vi "Autonomous Independent.vi"   [LabVIEW 2018]
doc: "This VI is called when autonomous begins, and will automatically be terminated when autonomous ends. You can carry out timed or sensor driven robot movement independently without needing to return to the caller."
uses:
  <vilib>/Rock Robotics/WPI/Utilities/WPI_GetSetVariantRefNum.vi
  <vilib>/Rock Robotics/Network Tables/NT Read String.vi
  Robot Global Data.vi
  <vilib>/Rock Robotics/WPI/RobotDrive/WPI_RobotDriveMecanumDrive_Cartesian.vi
panel:
  # "Be sure to right-click and choose Data Operations>>Make Current Value default if you want to save the array values with the VI"
types:
  T1 = typedef "WPI_RobotDriveDevRef.ctl" = cluster{"DevStatus":errorcluster, "Motors[]":T2[], "Square Inputs":bool, "Max Output":dbl}
  T2 = typedef "WPI_MotorControlDeviceRef.ctl" = cluster{"DeviceStatus":errorcluster, "Type":T3, "PWM":cluster{"PWM Channel":T4, "DeadBand":T5}, "CAN":cluster{"Device Number":u8, "SetOutput VI Ref":variant, "GetOutput VI Ref":variant, "Enable VI Ref":variant, "Disable VI Ref":variant, "Data":variant}, "Invert":bool, "DIO PWM":cluster{"PWM \"Enable\" Channel":T4, "DIOChannel":T6, "PWM Rate":dbl}}
  T3 = typedef "WPI_MotorControlType.ctl" = enum16{"PWM", "CAN", "DIO PWM"}
  T4 = typedef "FPGA_DIOPWMChannel.ctl" = enum8{"PWM 0", "PWM 1", "PWM 2", "PWM 3", "PWM 4", "PWM 5", "PWM 6", "PWM 7", "PWM 8", "PWM 9", "PWM MXP 0", "PWM MXP 1", "PWM MXP 2", "PWM MXP 3", "PWM MXP 4", "PWM MXP 5", "PWM MXP 6", "PWM MXP 7", "PWM MXP 8", "PWM MXP 9", "Invalid"}
  T5 = typedef "WPI_PWMDeadband.ctl" = cluster{"Name":string, "maxPositivePwm":i32, "minPositivePwm":i32, "centerPwm":i32, "maxNegativePwm":i32, "minNegativePwm":i32, "angularRange":u16}
  T6 = typedef "FPGA_DIOChannel.ctl" = enum8{"DIO 0", "DIO 1", "DIO 2", "DIO 3", "DIO 4", "DIO 5", "DIO 6", "DIO 7", "DIO 8", "DIO 9", "DIO MXP 0", "DIO MXP 1", "DIO MXP 2", "DIO MXP 3", "DIO MXP 4", "DIO MXP 5", "DIO MXP 6", "DIO MXP 7", "DIO MXP 8", "DIO MXP 9", "DIO MXP 10", "DIO MXP 11", "DIO MXP 12", "DIO MXP 13", "DIO MXP 14", "DIO MXP 15", "SPI Port CS1", "SPI Port CS2", "SPI Port CS3", "SPI Port MISO", "SPI Port MOSI", "Invalid"}
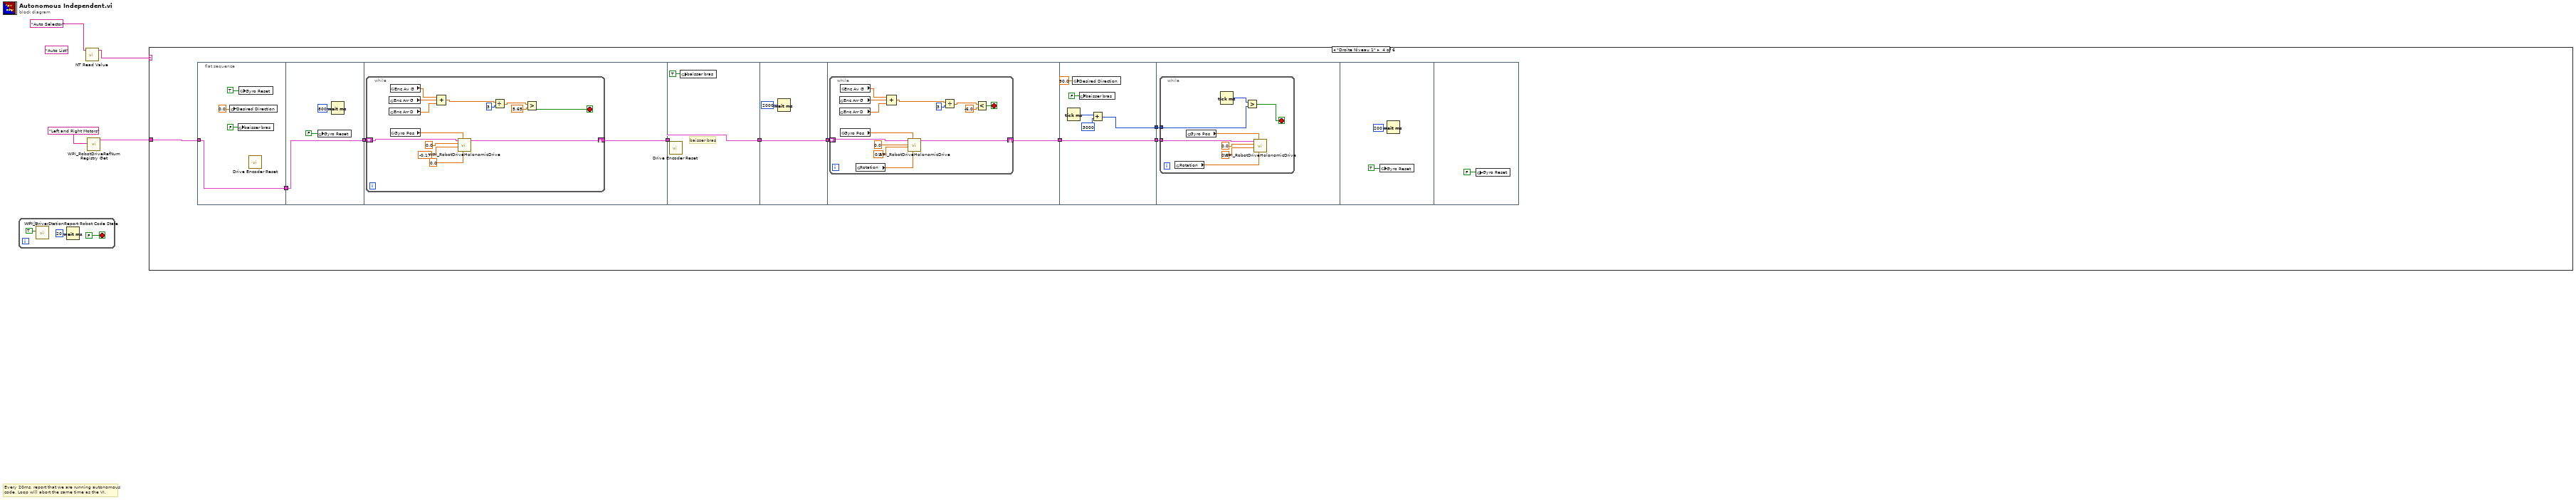
[diagram p0: block diagram]
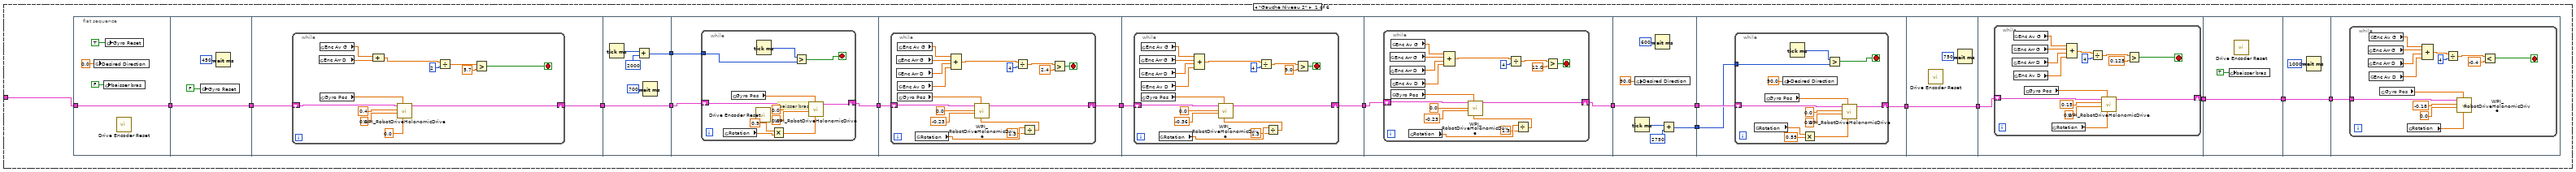
[diagram p2: hidden frame]
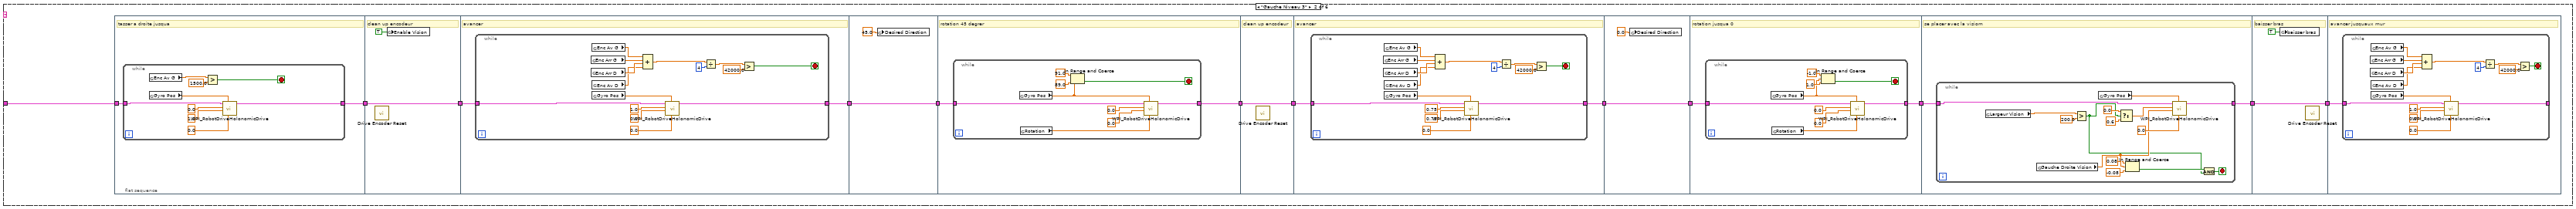
[diagram p3: hidden frame]
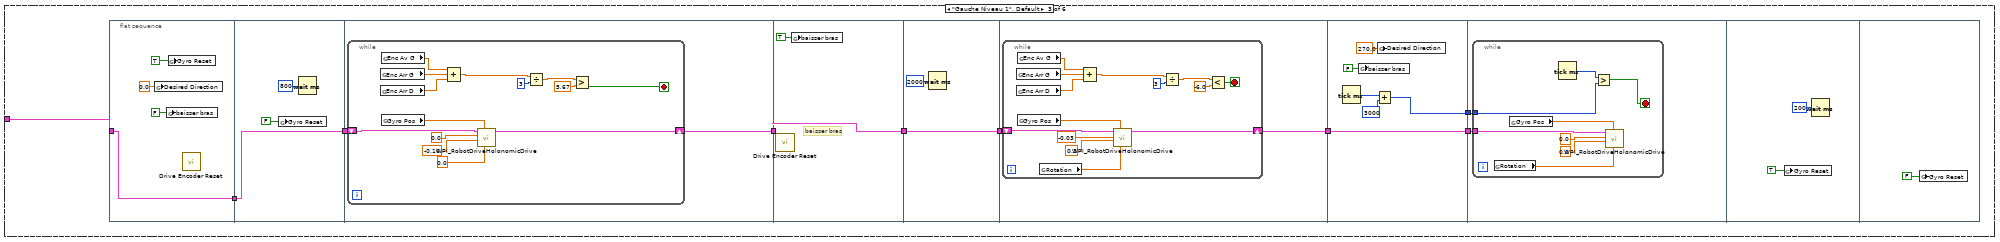
[diagram p4: hidden frame]
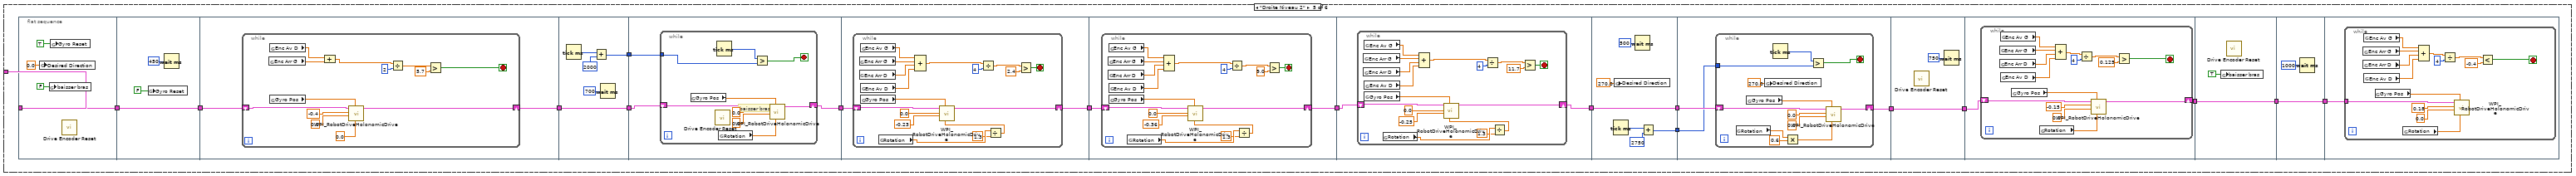
[diagram p5: hidden frame]
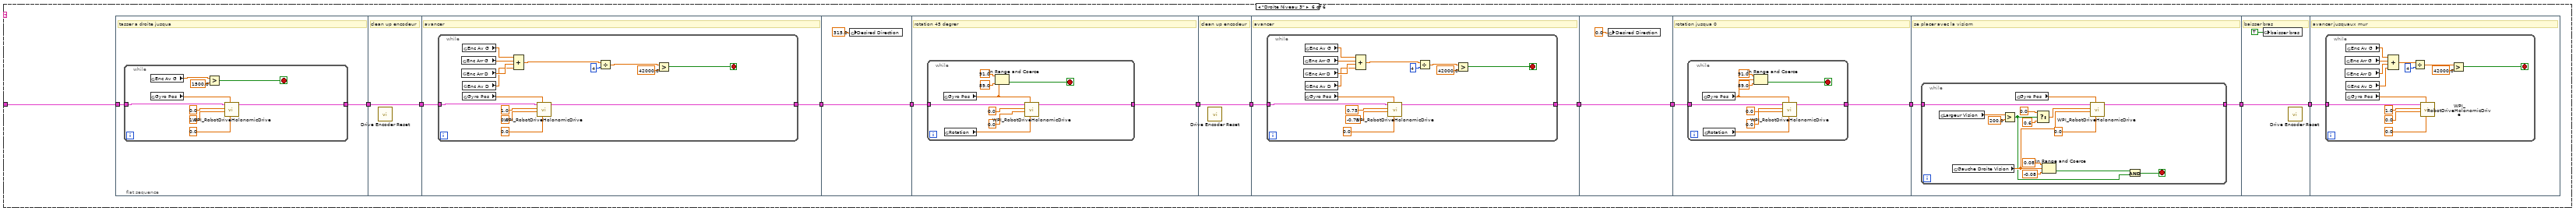
[diagram p6: hidden frame]
diagram:
  (unwired) "Auto List" ("Name")
  # "Every 20ms, report that we are running autonomous\ncode. Loop will abort the same time as the VI."
  n1 = while {
    stop <- FALSE stop-if-true
    n2 = call <vilib>:"WPI_DriverStationReport Robot Code State.vi"("Autonomous"=TRUE) -> ()  [unwired: 10 in, 1 out]
    n3 = Wait (ms)(milliseconds to wait=u32 20) -> ()  [unwired: 1 out]
  }
  n4 = call-poly <vilib>:"NT Read Value.vi"("Name"="Auto Selector") -> ("String"=w4:string)  [unwired: 9 in, 1 out]
  n5 = call <vilib>:"WPI_RobotDriveRefNum Registry Get.vi"("refnum name"="Left and Right Motors") -> ("RobotDriveDevRef"=w2:T1)  [unwired: 1 in, 9 out]
  n6 = case shown="\"Droite Niveau 1\"" w4 {
    tunnel: w2 -> [w8 w189 w303 w381 w459 w617]
    frame "Gauche Niveau 2" {
      n7 = flat-sequence {
        tunnel: w8 -> [w28]
        tunnel: [w28] -> w24
        tunnel: w24 -> [w29]
        tunnel: [w29] -> w23
        tunnel: [w33] -> w22
        tunnel: w23 -> [w32]
        tunnel: w22 -> [w51]
        tunnel: [w51] -> w21
        tunnel: [w48] -> w20
        tunnel: [w53] -> w19
        tunnel: w21 -> [w54]
        tunnel: w20 -> [w52]
        tunnel: w19 -> [w67]
        tunnel: [w66] -> w18
        tunnel: w18 -> [w86]
        tunnel: [w85] -> w17
        tunnel: w17 -> [w105]
        tunnel: [w104] -> w16
        tunnel: [w127] -> w15
        tunnel: w16 -> [w127]
        tunnel: [w123] -> w14
        tunnel: w15 -> [w131]
        tunnel: [w130] -> w13
        tunnel: w14 -> [w129]
        tunnel: w13 -> [w145]
        tunnel: [w145] -> w12
        tunnel: w12 -> [w147]
        tunnel: [w146] -> w11
        tunnel: w11 -> [w163]
        tunnel: [w163] -> w10
        tunnel: w10 -> [w166]
        tunnel: [w166] -> w9
        tunnel: w9 -> [w167]
        frame #0 {
          n8 = global write "Robot Global Data.vi" "Desired Direction"(0.0 ("Desired Direction")) -> ()
          n9 = global write "Robot Global Data.vi" "baisser bras"(FALSE) -> ()
          n10 = global write "Robot Global Data.vi" "Gyro Reset"(TRUE) -> ()
          n11 = call "Drive Encoder Reset.vi"() -> ()  [unwired: 12 in]
        }
        frame #1 {
          n12 = global write "Robot Global Data.vi" "Gyro Reset"(FALSE) -> ()
          n13 = Wait (ms)(milliseconds to wait=u32 450) -> ()  [unwired: 1 out]
        }
        frame #2 {
          n14 = while {
            shift-right: [w43] -> w33
            shift-left: w32 -> [w44]
            stop <- w38 stop-if-true
            n15 = global read "Robot Global Data.vi" "Enc Arr D"() -> (w36:dbl)
            n16 = global read "Robot Global Data.vi" "Enc Av G"() -> (w37:dbl)
            n17 = global read "Robot Global Data.vi" "Gyro Pos"() -> (w35:dbl)
            n18 = Compound Arithmetic op=ADD(w37, w36) -> (w42:dbl)
            n19 = call-poly <vilib>:"WPI_RobotDriveHolonomicDrive.vi"("Rotation"=0.0, "Gyro Angle"=w35, "Y"=0.0, "X"=0.4, "RobotDriveDevRef"=w44) -> ("RobotDriveDevRef"=w43:T1)  [unwired: 4 in, 2 out]
            n20 = Divide(x=w42, y=2) -> (x/y=w40:dbl)
            n21 = Greater?(x=w40, y=5.7) -> (0:w38:bool)
          }
        }
        frame #3 {
          n22 = Tick Count (ms)() -> (millisecond timer value=w50:u32)
          n23 = Add(x=w50, y=u32 2000) -> (x+y=w48:u32)
          n24 = Wait (ms)(milliseconds to wait=u32 700) -> ()  [unwired: 1 out]
        }
        frame #4 {
          # "baisser bras"
          n25 = while {
            shift-right: [w61] -> w53
            shift-left: w54 -> [w62]
            tunnel: w52 -> [w58]
            stop <- w59 stop-if-true
            n26 = global read "Robot Global Data.vi" "Rotation"() -> (w57:dbl)
            n27 = global read "Robot Global Data.vi" "Gyro Pos"() -> (w63:dbl)
            n28 = Tick Count (ms)() -> (millisecond timer value=w60:u32)
            n29 = Multiply(x=0.9, y=w57) -> (x*y=w55:dbl)
            n30 = Greater?(x=w60, y=w58) -> (0:w59:bool)
            n31 = call-poly <vilib>:"WPI_RobotDriveHolonomicDrive.vi"("Rotation"=w55, "Gyro Angle"=w63, "Y"=0.0, "X"=0.0, "RobotDriveDevRef"=w62) -> ("RobotDriveDevRef"=w61:T1)  [unwired: 4 in, 2 out]
          }
          n32 = call "Drive Encoder Reset.vi"() -> ()  [unwired: 12 in]
        }
        frame #5 {
          n33 = while {
            shift-right: [w82] -> w66
            shift-left: w67 -> [w83]
            stop <- w77 stop-if-true
            n34 = global read "Robot Global Data.vi" "Enc Arr G"() -> (w75:dbl)
            n35 = global read "Robot Global Data.vi" "Enc Arr D"() -> (w74:dbl)
            n36 = global read "Robot Global Data.vi" "Enc Av G"() -> (w76:dbl)
            n37 = global read "Robot Global Data.vi" "Enc Av D"() -> (w73:dbl)
            n38 = global read "Robot Global Data.vi" "Gyro Pos"() -> (w72:dbl)
            n39 = global read "Robot Global Data.vi" "Rotation"() -> (w70:dbl)
            n40 = Compound Arithmetic op=ADD(w76, w75, w74, w73) -> (w81:dbl)
            n41 = Divide(x=w81, y=4) -> (x/y=w79:dbl)
            n42 = Divide(x=w70, y=1.3) -> (x/y=w68:dbl)
            n43 = call-poly <vilib>:"WPI_RobotDriveHolonomicDrive.vi"("Rotation"=w68, "Gyro Angle"=w72, "Y"=-0.23, "X"=0.0, "RobotDriveDevRef"=w83) -> ("RobotDriveDevRef"=w82:T1)  [unwired: 4 in, 2 out]
            n44 = Greater?(x=w79, y=2.4) -> (0:w77:bool)
          }
        }
        frame #6 {
          n45 = while {
            shift-right: [w101] -> w85
            shift-left: w86 -> [w102]
            stop <- w96 stop-if-true
            n46 = global read "Robot Global Data.vi" "Enc Arr G"() -> (w94:dbl)
            n47 = global read "Robot Global Data.vi" "Enc Arr D"() -> (w93:dbl)
            n48 = global read "Robot Global Data.vi" "Enc Av G"() -> (w95:dbl)
            n49 = global read "Robot Global Data.vi" "Enc Av D"() -> (w92:dbl)
            n50 = global read "Robot Global Data.vi" "Gyro Pos"() -> (w91:dbl)
            n51 = global read "Robot Global Data.vi" "Rotation"() -> (w89:dbl)
            n52 = Compound Arithmetic op=ADD(w95, w94, w93, w92) -> (w100:dbl)
            n53 = Divide(x=w100, y=4) -> (x/y=w98:dbl)
            n54 = Divide(x=w89, y=1.3) -> (x/y=w87:dbl)
            n55 = call-poly <vilib>:"WPI_RobotDriveHolonomicDrive.vi"("Rotation"=w87, "Gyro Angle"=w91, "Y"=-0.36, "X"=0.0, "RobotDriveDevRef"=w102) -> ("RobotDriveDevRef"=w101:T1)  [unwired: 4 in, 2 out]
            n56 = Greater?(x=w98, y=9.0) -> (0:w96:bool)
          }
        }
        frame #7 {
          n57 = while {
            shift-right: [w120] -> w104
            shift-left: w105 -> [w121]
            stop <- w115 stop-if-true
            n58 = global read "Robot Global Data.vi" "Enc Arr G"() -> (w113:dbl)
            n59 = global read "Robot Global Data.vi" "Enc Arr D"() -> (w112:dbl)
            n60 = global read "Robot Global Data.vi" "Enc Av G"() -> (w114:dbl)
            n61 = global read "Robot Global Data.vi" "Enc Av D"() -> (w111:dbl)
            n62 = global read "Robot Global Data.vi" "Gyro Pos"() -> (w110:dbl)
            n63 = global read "Robot Global Data.vi" "Rotation"() -> (w108:dbl)
            n64 = Compound Arithmetic op=ADD(w114, w113, w112, w111) -> (w119:dbl)
            n65 = Divide(x=w119, y=4) -> (x/y=w117:dbl)
            n66 = Divide(x=w108, y=1.3) -> (x/y=w106:dbl)
            n67 = call-poly <vilib>:"WPI_RobotDriveHolonomicDrive.vi"("Rotation"=w106, "Gyro Angle"=w110, "Y"=-0.23, "X"=0.0, "RobotDriveDevRef"=w121) -> ("RobotDriveDevRef"=w120:T1)  [unwired: 4 in, 2 out]
            n68 = Greater?(x=w117, y=12.0) -> (0:w115:bool)
          }
        }
        frame #8 {
          n69 = Tick Count (ms)() -> (millisecond timer value=w125:u32)
          n70 = global write "Robot Global Data.vi" "Desired Direction"(90.0 ("Desired Direction")) -> ()
          n71 = Wait (ms)(milliseconds to wait=u32 600) -> ()  [unwired: 1 out]
          n72 = Add(x=w125, y=u32 2750) -> (x+y=w123:u32)
        }
        frame #9 {
          n73 = while {
            tunnel: w129 -> [w136]
            shift-right: [w139] -> w130
            shift-left: w131 -> [w140]
            stop <- w137 stop-if-true
            n74 = global read "Robot Global Data.vi" "Rotation"() -> (w135:dbl)
            n75 = global read "Robot Global Data.vi" "Gyro Pos"() -> (w141:dbl)
            n76 = global write "Robot Global Data.vi" "Desired Direction"(90.0 ("Desired Direction")) -> ()
            n77 = Tick Count (ms)() -> (millisecond timer value=w138:u32)
            n78 = Multiply(x=w135, y=0.55) -> (x*y=w134:dbl)
            n79 = Greater?(x=w138, y=w136) -> (0:w137:bool)
            n80 = call-poly <vilib>:"WPI_RobotDriveHolonomicDrive.vi"("Rotation"=w134, "Gyro Angle"=w141, "Y"=0.0, "X"=0.0, "RobotDriveDevRef"=w140) -> ("RobotDriveDevRef"=w139:T1)  [unwired: 4 in, 2 out]
          }
        }
        frame #10 {
          n81 = call "Drive Encoder Reset.vi"() -> ()  [unwired: 12 in]
          n82 = Wait (ms)(milliseconds to wait=u32 750) -> ()  [unwired: 1 out]
        }
        frame #11 {
          n83 = while {
            shift-right: [w148] -> w146
            shift-left: w147 -> [w158]
            stop <- w149 stop-if-true
            n84 = global read "Robot Global Data.vi" "Enc Arr G"() -> (w152:dbl)
            n85 = global read "Robot Global Data.vi" "Enc Arr D"() -> (w151:dbl)
            n86 = global read "Robot Global Data.vi" "Enc Av G"() -> (w153:dbl)
            n87 = global read "Robot Global Data.vi" "Enc Av D"() -> (w150:dbl)
            n88 = global read "Robot Global Data.vi" "Gyro Pos"() -> (w160:dbl)
            n89 = global read "Robot Global Data.vi" "Rotation"() -> (w159:dbl)
            n90 = Compound Arithmetic op=ADD(w153, w152, w151, w150) -> (w157:dbl)
            n91 = Divide(x=w157, y=4) -> (x/y=w155:dbl)
            n92 = call-poly <vilib>:"WPI_RobotDriveHolonomicDrive.vi"("Rotation"=w159, "Gyro Angle"=w160, "Y"=0.0, "X"=0.15, "RobotDriveDevRef"=w158) -> ("RobotDriveDevRef"=w148:T1)  [unwired: 4 in, 2 out]
            n93 = Greater?(x=w155, y=0.125) -> (0:w149:bool)
          }
        }
        frame #12 {
          n94 = global write "Robot Global Data.vi" "baisser bras"(TRUE) -> ()
          n95 = call "Drive Encoder Reset.vi"() -> ()  [unwired: 12 in]
        }
        frame #13 {
          n96 = Wait (ms)(milliseconds to wait=u32 1000) -> ()  [unwired: 1 out]
        }
        frame #14 {
          n97 = while {
            tunnel: w167 -> [w177]
            stop <- w168 stop-if-true
            n98 = global read "Robot Global Data.vi" "Enc Arr G"() -> (w171:dbl)
            n99 = global read "Robot Global Data.vi" "Enc Arr D"() -> (w170:dbl)
            n100 = global read "Robot Global Data.vi" "Enc Av G"() -> (w172:dbl)
            n101 = global read "Robot Global Data.vi" "Enc Av D"() -> (w169:dbl)
            n102 = global read "Robot Global Data.vi" "Gyro Pos"() -> (w179:dbl)
            n103 = global read "Robot Global Data.vi" "Rotation"() -> (w178:dbl)
            n104 = Compound Arithmetic op=ADD(w172, w171, w170, w169) -> (w176:dbl)
            n105 = Divide(x=w176, y=4) -> (x/y=w174:dbl)
            n106 = call-poly <vilib>:"WPI_RobotDriveHolonomicDrive.vi"("Rotation"=w178, "Gyro Angle"=w179, "Y"=0.0, "X"=-0.18, "RobotDriveDevRef"=w177) -> ()  [unwired: 4 in, 3 out]
            n107 = Less?(x=w174, y=-0.4) -> (x < y?=w168:bool)
          }
        }
      }
    }
    frame "Gauche Niveau 3" {
      n108 = flat-sequence {
        tunnel: [w195] -> w193
        tunnel: w189 -> [w194]
        tunnel: w193 -> [w206]
        tunnel: [w206] -> w192
        tunnel: w192 -> [w208]
        tunnel: [w207] -> w191
        tunnel: w191 -> [w225]
        tunnel: [w225] -> w190
        tunnel: w190 -> [w227]
        tunnel: [w226] -> w188
        tunnel: w188 -> [w237]
        tunnel: [w237] -> w187
        tunnel: w187 -> [w239]
        tunnel: [w238] -> w186
        tunnel: w186 -> [w255]
        tunnel: [w255] -> w185
        tunnel: w185 -> [w258]
        tunnel: [w257] -> w184
        tunnel: w184 -> [w269]
        tunnel: [w268] -> w183
        tunnel: w183 -> [w286]
        tunnel: [w286] -> w182
        tunnel: w182 -> [w287]
        frame #0 {
          # "tasser a droite jusqua"
          n109 = while {
            tunnel: [w204] -> w195
            tunnel: w194 -> [w200]
            stop <- w197 stop-if-true
            n110 = global read "Robot Global Data.vi" "Enc Av G"() -> (w198:dbl)
            n111 = global read "Robot Global Data.vi" "Gyro Pos"() -> (w196:dbl)
            n112 = Greater?(x=w198, y=1500.0) -> (0:w197:bool)
            n113 = call-poly <vilib>:"WPI_RobotDriveHolonomicDrive.vi"("Rotation"=0.0, "Gyro Angle"=w196, "Y"=1.0, "X"=0.0, "RobotDriveDevRef"=w200) -> ("RobotDriveDevRef"=w204:T1)  [unwired: 4 in, 2 out]
          }
        }
        frame #1 {
          # "clean up encodeur"
          n114 = call "Drive Encoder Reset.vi"() -> ()  [unwired: 12 in]
          n115 = global write "Robot Global Data.vi" "Enable Vision"(TRUE ("Enable Vision")) -> ()
        }
        frame #2 {
          # "avancer"
          n116 = while {
            tunnel: w208 -> [w223]
            tunnel: [w222] -> w207
            stop <- w214 stop-if-true
            n117 = global read "Robot Global Data.vi" "Enc Arr G"() -> (w212:dbl)
            n118 = global read "Robot Global Data.vi" "Enc Arr D"() -> (w211:dbl)
            n119 = global read "Robot Global Data.vi" "Enc Av G"() -> (w213:dbl)
            n120 = global read "Robot Global Data.vi" "Enc Av D"() -> (w210:dbl)
            n121 = global read "Robot Global Data.vi" "Gyro Pos"() -> (w209:dbl)
            n122 = Compound Arithmetic op=ADD(w213, w212, w211, w210) -> (w218:dbl)
            n123 = call-poly <vilib>:"WPI_RobotDriveHolonomicDrive.vi"("Rotation"=0.0, "Gyro Angle"=w209, "Y"=0.0, "X"=1.0, "RobotDriveDevRef"=w223) -> ("RobotDriveDevRef"=w222:T1)  [unwired: 4 in, 2 out]
            n124 = Divide(x=w218, y=4) -> (x/y=w216:dbl)
            n125 = Greater?(x=w216, y=42000.0) -> (0:w214:bool)
          }
        }
        frame #3 {
          n126 = global write "Robot Global Data.vi" "Desired Direction"(45.0 ("Desired Direction")) -> ()
        }
        frame #4 {
          # "rotation 45 degrer"
          n127 = while {
            tunnel: [w234] -> w226
            tunnel: w227 -> [w230]
            stop <- w228 stop-if-true
            n128 = global read "Robot Global Data.vi" "Gyro Pos"() -> (w229:dbl)
            n129 = global read "Robot Global Data.vi" "Rotation"() -> (w231:dbl)
            n130 = In Range and Coerce(upper limit=91.0, x=w229, lower limit=89.0) -> (In Range?=w228:bool)  [unwired: 1 out]
            n131 = call-poly <vilib>:"WPI_RobotDriveHolonomicDrive.vi"("Rotation"=w231, "Gyro Angle"=w229, "Y"=0.0, "X"=0.0, "RobotDriveDevRef"=w230) -> ("RobotDriveDevRef"=w234:T1)  [unwired: 4 in, 2 out]
          }
        }
        frame #5 {
          # "clean up encodeur"
          n132 = call "Drive Encoder Reset.vi"() -> ()  [unwired: 12 in]
        }
        frame #6 {
          # "avancer"
          n133 = while {
            tunnel: [w254] -> w238
            tunnel: w239 -> [w245]
            stop <- w246 stop-if-true
            n134 = global read "Robot Global Data.vi" "Enc Arr G"() -> (w243:dbl)
            n135 = global read "Robot Global Data.vi" "Enc Arr D"() -> (w242:dbl)
            n136 = global read "Robot Global Data.vi" "Enc Av G"() -> (w240:dbl)
            n137 = global read "Robot Global Data.vi" "Enc Av D"() -> (w241:dbl)
            n138 = global read "Robot Global Data.vi" "Gyro Pos"() -> (w244:dbl)
            n139 = Compound Arithmetic op=ADD(w240, w243, w242, w241) -> (w250:dbl)
            n140 = call-poly <vilib>:"WPI_RobotDriveHolonomicDrive.vi"("Rotation"=0.0, "Gyro Angle"=w244, "Y"=0.75, "X"=0.75, "RobotDriveDevRef"=w245) -> ("RobotDriveDevRef"=w254:T1)  [unwired: 4 in, 2 out]
            n141 = Divide(x=w250, y=4) -> (x/y=w248:dbl)
            n142 = Greater?(x=w248, y=42000.0) -> (0:w246:bool)
          }
        }
        frame #7 {
          n143 = global write "Robot Global Data.vi" "Desired Direction"(0.0 ("Desired Direction")) -> ()
        }
        frame #8 {
          # "rotation jusqua 0"
          n144 = while {
            tunnel: [w265] -> w257
            tunnel: w258 -> [w260]
            stop <- w262 stop-if-true
            n145 = global read "Robot Global Data.vi" "Gyro Pos"() -> (w259:dbl)
            n146 = global read "Robot Global Data.vi" "Rotation"() -> (w261:dbl)
            n147 = In Range and Coerce(upper limit=-1.0, x=w259, lower limit=1.0) -> (In Range?=w262:bool)  [unwired: 1 out]
            n148 = call-poly <vilib>:"WPI_RobotDriveHolonomicDrive.vi"("Rotation"=w261, "Gyro Angle"=w259, "Y"=0.0, "X"=0.0, "RobotDriveDevRef"=w260) -> ("RobotDriveDevRef"=w265:T1)  [unwired: 4 in, 2 out]
          }
        }
        frame #9 {
          # "se placer avec la visiom"
          n149 = while {
            tunnel: [w284] -> w268
            tunnel: w269 -> [w281]
            stop <- w282 stop-if-true
            n150 = global read "Robot Global Data.vi" "Largeur Vision"() -> (w276:dbl)
            n151 = global read "Robot Global Data.vi" "Gauche Droite Vision"() -> (w280:dbl)
            n152 = Greater?(x=w276, y=200.0) -> (0:w271:bool)
            n153 = global read "Robot Global Data.vi" "Gyro Pos"() -> (w270:dbl)
            n154 = Select(t=0.0, s=w271, f=0.6) -> (s? t:f=w274:dbl)
            n155 = In Range and Coerce(upper limit=0.08, x=w280, lower limit=-0.08) -> (In Range?=w277:bool)  [unwired: 1 out]
            n156 = call-poly <vilib>:"WPI_RobotDriveHolonomicDrive.vi"("Rotation"=0.0, "Gyro Angle"=w270, "Y"=w280, "X"=w274, "RobotDriveDevRef"=w281) -> ("RobotDriveDevRef"=w284:T1)  [unwired: 4 in, 2 out]
            n157 = And(x=w277, y=w271) -> (x .and. y?=w282:bool)
          }
        }
        frame #10 {
          # "baisser bras"
          n158 = global write "Robot Global Data.vi" "baisser bras"(TRUE) -> ()
          n159 = call "Drive Encoder Reset.vi"() -> ()  [unwired: 12 in]
        }
        frame #11 {
          # "avancer jusquaux mur"
          n160 = while {
            tunnel: w287 -> [w302]
            tunnel: [w301] -> _
            stop <- w293 stop-if-true
            n161 = global read "Robot Global Data.vi" "Enc Arr G"() -> (w291:dbl)
            n162 = global read "Robot Global Data.vi" "Enc Arr D"() -> (w289:dbl)
            n163 = global read "Robot Global Data.vi" "Enc Av G"() -> (w290:dbl)
            n164 = global read "Robot Global Data.vi" "Enc Av D"() -> (w288:dbl)
            n165 = global read "Robot Global Data.vi" "Gyro Pos"() -> (w292:dbl)
            n166 = Compound Arithmetic op=ADD(w290, w291, w289, w288) -> (w297:dbl)
            n167 = call-poly <vilib>:"WPI_RobotDriveHolonomicDrive.vi"("Rotation"=0.0, "Gyro Angle"=w292, "Y"=0.0, "X"=1.0, "RobotDriveDevRef"=w302) -> ("RobotDriveDevRef"=w301:T1)  [unwired: 4 in, 2 out]
            n168 = Divide(x=w297, y=4) -> (x/y=w295:dbl)
            n169 = Greater?(x=w295, y=42000.0) -> (0:w293:bool)
          }
        }
      }
    }
    frame "Gauche Niveau 1", Default {
      n170 = flat-sequence {
        tunnel: w303 -> [w315]
        tunnel: [w315] -> w311
        tunnel: w311 -> [w318]
        tunnel: [w318] -> w310
        tunnel: [w319] -> w309
        tunnel: w310 -> [w320]
        tunnel: [w336] -> w308
        tunnel: w309 -> [w336]
        tunnel: w308 -> [w338]
        tunnel: [w338] -> w307
        tunnel: w307 -> [w340]
        tunnel: [w339] -> w306
        tunnel: [w359] -> w305
        tunnel: w306 -> [w359]
        tunnel: [w355] -> w304
        tunnel: w305 -> [w362]
        tunnel: w304 -> [w361]
        frame #0 {
          n171 = global write "Robot Global Data.vi" "Desired Direction"(0.0 ("Desired Direction")) -> ()
          n172 = global write "Robot Global Data.vi" "baisser bras"(FALSE) -> ()
          n173 = global write "Robot Global Data.vi" "Gyro Reset"(TRUE) -> ()
          n174 = call "Drive Encoder Reset.vi"() -> ()  [unwired: 12 in]
        }
        frame #1 {
          n175 = global write "Robot Global Data.vi" "Gyro Reset"(FALSE) -> ()
          n176 = Wait (ms)(milliseconds to wait=u32 800) -> ()  [unwired: 1 out]
        }
        frame #2 {
          n177 = while {
            shift-right: [w332] -> w319
            shift-left: w320 -> [w333]
            stop <- w327 stop-if-true
            n178 = global read "Robot Global Data.vi" "Enc Arr G"() -> (w325:dbl)
            n179 = global read "Robot Global Data.vi" "Enc Arr D"() -> (w324:dbl)
            n180 = global read "Robot Global Data.vi" "Enc Av G"() -> (w326:dbl)
            n181 = global read "Robot Global Data.vi" "Gyro Pos"() -> (w323:dbl)
            n182 = Compound Arithmetic op=ADD(w326, w325, w324) -> (w331:dbl)
            n183 = call-poly <vilib>:"WPI_RobotDriveHolonomicDrive.vi"("Rotation"=0.0, "Gyro Angle"=w323, "Y"=-0.16, "X"=0.0, "RobotDriveDevRef"=w333) -> ("RobotDriveDevRef"=w332:T1)  [unwired: 4 in, 2 out]
            n184 = Divide(x=w331, y=3) -> (x/y=w329:dbl)
            n185 = Greater?(x=w329, y=5.67) -> (0:w327:bool)
          }
        }
        frame #3 {
          # "baisser bras"
          n186 = call "Drive Encoder Reset.vi"() -> ()  [unwired: 12 in]
          n187 = global write "Robot Global Data.vi" "baisser bras"(TRUE) -> ()
        }
        frame #4 {
          n188 = Wait (ms)(milliseconds to wait=u32 2000) -> ()  [unwired: 1 out]
        }
        frame #5 {
          n189 = while {
            shift-right: [w352] -> w339
            shift-left: w340 -> [w353]
            stop <- w347 stop-if-true
            n190 = global read "Robot Global Data.vi" "Enc Arr G"() -> (w345:dbl)
            n191 = global read "Robot Global Data.vi" "Enc Arr D"() -> (w344:dbl)
            n192 = global read "Robot Global Data.vi" "Enc Av G"() -> (w346:dbl)
            n193 = global read "Robot Global Data.vi" "Gyro Pos"() -> (w343:dbl)
            n194 = global read "Robot Global Data.vi" "Rotation"() -> (w342:dbl)
            n195 = Compound Arithmetic op=ADD(w346, w345, w344) -> (w351:dbl)
            n196 = call-poly <vilib>:"WPI_RobotDriveHolonomicDrive.vi"("Rotation"=w342, "Gyro Angle"=w343, "Y"=0.3, "X"=-0.03, "RobotDriveDevRef"=w353) -> ("RobotDriveDevRef"=w352:T1)  [unwired: 4 in, 2 out]
            n197 = Divide(x=w351, y=3) -> (x/y=w349:dbl)
            n198 = Less?(x=w349, y=-6.0) -> (x < y?=w347:bool)
          }
        }
        frame #6 {
          n199 = Tick Count (ms)() -> (millisecond timer value=w357:u32)
          n200 = global write "Robot Global Data.vi" "baisser bras"(FALSE) -> ()
          n201 = Add(x=w357, y=u32 3000) -> (x+y=w355:u32)
          n202 = global write "Robot Global Data.vi" "Desired Direction"(270.0 ("Desired Direction")) -> ()
        }
        frame #7 {
          n203 = while {
            tunnel: w362 -> [w367]
            tunnel: w361 -> [w364]
            stop <- w363 stop-if-true
            n204 = global read "Robot Global Data.vi" "Rotation"() -> (w368:dbl)
            n205 = global read "Robot Global Data.vi" "Gyro Pos"() -> (w366:dbl)
            n206 = Tick Count (ms)() -> (millisecond timer value=w365:u32)
            n207 = Greater?(x=w365, y=w364) -> (0:w363:bool)
            n208 = call-poly <vilib>:"WPI_RobotDriveHolonomicDrive.vi"("Rotation"=w368, "Gyro Angle"=w366, "Y"=0.0, "X"=0.0, "RobotDriveDevRef"=w367) -> ()  [unwired: 4 in, 3 out]
          }
        }
        frame #8 {
          n209 = global write "Robot Global Data.vi" "Gyro Reset"(TRUE) -> ()
          n210 = Wait (ms)(milliseconds to wait=u32 200) -> ()  [unwired: 1 out]
        }
        frame #9 {
          n211 = global write "Robot Global Data.vi" "Gyro Reset"(FALSE) -> ()
        }
      }
    }
    frame "Droite Niveau 1" {
      n212 = flat-sequence {
        tunnel: w381 -> [w386]
        tunnel: [w386] -> w376
        tunnel: w376 -> [w389]
        tunnel: [w389] -> w374
        tunnel: [w390] -> w382
        tunnel: w374 -> [w391]
        tunnel: [w407] -> w380
        tunnel: w382 -> [w407]
        tunnel: w380 -> [w409]
        tunnel: [w409] -> w379
        tunnel: w379 -> [w411]
        tunnel: [w410] -> w377
        tunnel: [w430] -> w378
        tunnel: w377 -> [w430]
        tunnel: [w426] -> w375
        tunnel: w378 -> [w433]
        tunnel: w375 -> [w432]
        frame #0 {
          n213 = global write "Robot Global Data.vi" "Desired Direction"(0.0 ("Desired Direction")) -> ()
          n214 = global write "Robot Global Data.vi" "baisser bras"(FALSE) -> ()
          n215 = global write "Robot Global Data.vi" "Gyro Reset"(TRUE) -> ()
          n216 = call "Drive Encoder Reset.vi"() -> ()  [unwired: 12 in]
        }
        frame #1 {
          n217 = global write "Robot Global Data.vi" "Gyro Reset"(FALSE) -> ()
          n218 = Wait (ms)(milliseconds to wait=u32 800) -> ()  [unwired: 1 out]
        }
        frame #2 {
          n219 = while {
            shift-right: [w403] -> w390
            shift-left: w391 -> [w404]
            stop <- w398 stop-if-true
            n220 = global read "Robot Global Data.vi" "Enc Arr G"() -> (w396:dbl)
            n221 = global read "Robot Global Data.vi" "Enc Arr D"() -> (w395:dbl)
            n222 = global read "Robot Global Data.vi" "Enc Av G"() -> (w397:dbl)
            n223 = global read "Robot Global Data.vi" "Gyro Pos"() -> (w394:dbl)
            n224 = Compound Arithmetic op=ADD(w397, w396, w395) -> (w402:dbl)
            n225 = call-poly <vilib>:"WPI_RobotDriveHolonomicDrive.vi"("Rotation"=0.0, "Gyro Angle"=w394, "Y"=-0.17, "X"=0.0, "RobotDriveDevRef"=w404) -> ("RobotDriveDevRef"=w403:T1)  [unwired: 4 in, 2 out]
            n226 = Divide(x=w402, y=3) -> (x/y=w400:dbl)
            n227 = Greater?(x=w400, y=5.65) -> (0:w398:bool)
          }
        }
        frame #3 {
          # "baisser bras"
          n228 = call "Drive Encoder Reset.vi"() -> ()  [unwired: 12 in]
          n229 = global write "Robot Global Data.vi" "baisser bras"(TRUE) -> ()
        }
        frame #4 {
          n230 = Wait (ms)(milliseconds to wait=u32 2000) -> ()  [unwired: 1 out]
        }
        frame #5 {
          n231 = while {
            shift-right: [w423] -> w410
            shift-left: w411 -> [w424]
            stop <- w418 stop-if-true
            n232 = global read "Robot Global Data.vi" "Enc Arr G"() -> (w416:dbl)
            n233 = global read "Robot Global Data.vi" "Enc Arr D"() -> (w415:dbl)
            n234 = global read "Robot Global Data.vi" "Enc Av G"() -> (w417:dbl)
            n235 = global read "Robot Global Data.vi" "Gyro Pos"() -> (w414:dbl)
            n236 = global read "Robot Global Data.vi" "Rotation"() -> (w413:dbl)
            n237 = Compound Arithmetic op=ADD(w417, w416, w415) -> (w422:dbl)
            n238 = call-poly <vilib>:"WPI_RobotDriveHolonomicDrive.vi"("Rotation"=w413, "Gyro Angle"=w414, "Y"=0.3, "X"=0.0, "RobotDriveDevRef"=w424) -> ("RobotDriveDevRef"=w423:T1)  [unwired: 4 in, 2 out]
            n239 = Divide(x=w422, y=3) -> (x/y=w420:dbl)
            n240 = Less?(x=w420, y=-6.0) -> (x < y?=w418:bool)
          }
        }
        frame #6 {
          n241 = Tick Count (ms)() -> (millisecond timer value=w428:u32)
          n242 = global write "Robot Global Data.vi" "Desired Direction"(90.0 ("Desired Direction")) -> ()
          n243 = global write "Robot Global Data.vi" "baisser bras"(FALSE) -> ()
          n244 = Add(x=w428, y=u32 3000) -> (x+y=w426:u32)
        }
        frame #7 {
          n245 = while {
            tunnel: w433 -> [w438]
            tunnel: w432 -> [w435]
            stop <- w434 stop-if-true
            n246 = global read "Robot Global Data.vi" "Rotation"() -> (w439:dbl)
            n247 = global read "Robot Global Data.vi" "Gyro Pos"() -> (w437:dbl)
            n248 = Tick Count (ms)() -> (millisecond timer value=w436:u32)
            n249 = Greater?(x=w436, y=w435) -> (0:w434:bool)
            n250 = call-poly <vilib>:"WPI_RobotDriveHolonomicDrive.vi"("Rotation"=w439, "Gyro Angle"=w437, "Y"=0.0, "X"=0.0, "RobotDriveDevRef"=w438) -> ()  [unwired: 4 in, 3 out]
          }
        }
        frame #8 {
          n251 = global write "Robot Global Data.vi" "Gyro Reset"(TRUE) -> ()
          n252 = Wait (ms)(milliseconds to wait=u32 200) -> ()  [unwired: 1 out]
        }
        frame #9 {
          n253 = global write "Robot Global Data.vi" "Gyro Reset"(FALSE) -> ()
        }
      }
    }
    frame "Droite Niveau 2" {
      n254 = flat-sequence {
        tunnel: w459 -> [w465]
        tunnel: [w465] -> w461
        tunnel: w461 -> [w466]
        tunnel: [w466] -> w454
        tunnel: [w470] -> w453
        tunnel: w454 -> [w469]
        tunnel: w453 -> [w488]
        tunnel: [w488] -> w452
        tunnel: [w485] -> w451
        tunnel: [w490] -> w448
        tunnel: w452 -> [w491]
        tunnel: w451 -> [w489]
        tunnel: w448 -> [w502]
        tunnel: [w501] -> w447
        tunnel: w447 -> [w521]
        tunnel: [w520] -> w446
        tunnel: w446 -> [w540]
        tunnel: [w539] -> w445
        tunnel: [w562] -> w460
        tunnel: w445 -> [w562]
        tunnel: [w558] -> w456
        tunnel: w460 -> [w566]
        tunnel: [w565] -> w458
        tunnel: w456 -> [w564]
        tunnel: w458 -> [w580]
        tunnel: [w580] -> w457
        tunnel: w457 -> [w582]
        tunnel: [w581] -> w455
        tunnel: w455 -> [w598]
        tunnel: [w598] -> w450
        tunnel: w450 -> [w601]
        tunnel: [w601] -> w449
        tunnel: w449 -> [w602]
        frame #0 {
          n255 = global write "Robot Global Data.vi" "Desired Direction"(0.0 ("Desired Direction")) -> ()
          n256 = global write "Robot Global Data.vi" "baisser bras"(FALSE) -> ()
          n257 = global write "Robot Global Data.vi" "Gyro Reset"(TRUE) -> ()
          n258 = call "Drive Encoder Reset.vi"() -> ()  [unwired: 12 in]
        }
        frame #1 {
          n259 = global write "Robot Global Data.vi" "Gyro Reset"(FALSE) -> ()
          n260 = Wait (ms)(milliseconds to wait=u32 450) -> ()  [unwired: 1 out]
        }
        frame #2 {
          n261 = while {
            shift-right: [w480] -> w470
            shift-left: w469 -> [w481]
            stop <- w475 stop-if-true
            n262 = global read "Robot Global Data.vi" "Enc Arr G"() -> (w473:dbl)
            n263 = global read "Robot Global Data.vi" "Enc Av D"() -> (w474:dbl)
            n264 = global read "Robot Global Data.vi" "Gyro Pos"() -> (w472:dbl)
            n265 = Compound Arithmetic op=ADD(w474, w473) -> (w479:dbl)
            n266 = call-poly <vilib>:"WPI_RobotDriveHolonomicDrive.vi"("Rotation"=0.0, "Gyro Angle"=w472, "Y"=0.0, "X"=-0.4, "RobotDriveDevRef"=w481) -> ("RobotDriveDevRef"=w480:T1)  [unwired: 4 in, 2 out]
            n267 = Divide(x=w479, y=2) -> (x/y=w477:dbl)
            n268 = Greater?(x=w477, y=5.7) -> (0:w475:bool)
          }
        }
        frame #3 {
          n269 = Tick Count (ms)() -> (millisecond timer value=w487:u32)
          n270 = Add(x=w487, y=u32 2000) -> (x+y=w485:u32)
          n271 = Wait (ms)(milliseconds to wait=u32 700) -> ()  [unwired: 1 out]
        }
        frame #4 {
          # "baisser bras"
          n272 = while {
            shift-right: [w495] -> w490
            shift-left: w491 -> [w496]
            tunnel: w489 -> [w492]
            stop <- w493 stop-if-true
            n273 = global read "Robot Global Data.vi" "Gyro Pos"() -> (w498:dbl)
            n274 = Tick Count (ms)() -> (millisecond timer value=w494:u32)
            n275 = global read "Robot Global Data.vi" "Rotation"() -> (w497:dbl)
            n276 = Greater?(x=w494, y=w492) -> (0:w493:bool)
            n277 = call-poly <vilib>:"WPI_RobotDriveHolonomicDrive.vi"("Rotation"=w497, "Gyro Angle"=w498, "Y"=0.0, "X"=0.0, "RobotDriveDevRef"=w496) -> ("RobotDriveDevRef"=w495:T1)  [unwired: 4 in, 2 out]
          }
          n278 = call "Drive Encoder Reset.vi"() -> ()  [unwired: 12 in]
        }
        frame #5 {
          n279 = while {
            shift-right: [w517] -> w501
            shift-left: w502 -> [w518]
            stop <- w512 stop-if-true
            n280 = global read "Robot Global Data.vi" "Enc Arr G"() -> (w510:dbl)
            n281 = global read "Robot Global Data.vi" "Enc Arr D"() -> (w509:dbl)
            n282 = global read "Robot Global Data.vi" "Enc Av G"() -> (w511:dbl)
            n283 = global read "Robot Global Data.vi" "Enc Av D"() -> (w508:dbl)
            n284 = global read "Robot Global Data.vi" "Gyro Pos"() -> (w507:dbl)
            n285 = global read "Robot Global Data.vi" "Rotation"() -> (w505:dbl)
            n286 = Compound Arithmetic op=ADD(w511, w510, w509, w508) -> (w516:dbl)
            n287 = Divide(x=w516, y=4) -> (x/y=w514:dbl)
            n288 = Divide(x=w505, y=1.3) -> (x/y=w503:dbl)
            n289 = call-poly <vilib>:"WPI_RobotDriveHolonomicDrive.vi"("Rotation"=w503, "Gyro Angle"=w507, "Y"=-0.23, "X"=0.0, "RobotDriveDevRef"=w518) -> ("RobotDriveDevRef"=w517:T1)  [unwired: 4 in, 2 out]
            n290 = Greater?(x=w514, y=2.4) -> (0:w512:bool)
          }
        }
        frame #6 {
          n291 = while {
            shift-right: [w536] -> w520
            shift-left: w521 -> [w537]
            stop <- w531 stop-if-true
            n292 = global read "Robot Global Data.vi" "Enc Arr G"() -> (w529:dbl)
            n293 = global read "Robot Global Data.vi" "Enc Arr D"() -> (w528:dbl)
            n294 = global read "Robot Global Data.vi" "Enc Av G"() -> (w530:dbl)
            n295 = global read "Robot Global Data.vi" "Enc Av D"() -> (w527:dbl)
            n296 = global read "Robot Global Data.vi" "Gyro Pos"() -> (w526:dbl)
            n297 = global read "Robot Global Data.vi" "Rotation"() -> (w524:dbl)
            n298 = Compound Arithmetic op=ADD(w530, w529, w528, w527) -> (w535:dbl)
            n299 = Divide(x=w535, y=4) -> (x/y=w533:dbl)
            n300 = Divide(x=w524, y=1.3) -> (x/y=w522:dbl)
            n301 = call-poly <vilib>:"WPI_RobotDriveHolonomicDrive.vi"("Rotation"=w522, "Gyro Angle"=w526, "Y"=-0.36, "X"=0.0, "RobotDriveDevRef"=w537) -> ("RobotDriveDevRef"=w536:T1)  [unwired: 4 in, 2 out]
            n302 = Greater?(x=w533, y=9.0) -> (0:w531:bool)
          }
        }
        frame #7 {
          n303 = while {
            shift-right: [w555] -> w539
            shift-left: w540 -> [w556]
            stop <- w550 stop-if-true
            n304 = global read "Robot Global Data.vi" "Enc Arr G"() -> (w548:dbl)
            n305 = global read "Robot Global Data.vi" "Enc Arr D"() -> (w547:dbl)
            n306 = global read "Robot Global Data.vi" "Enc Av G"() -> (w549:dbl)
            n307 = global read "Robot Global Data.vi" "Enc Av D"() -> (w546:dbl)
            n308 = global read "Robot Global Data.vi" "Gyro Pos"() -> (w545:dbl)
            n309 = global read "Robot Global Data.vi" "Rotation"() -> (w543:dbl)
            n310 = Compound Arithmetic op=ADD(w549, w548, w547, w546) -> (w554:dbl)
            n311 = Divide(x=w554, y=4) -> (x/y=w552:dbl)
            n312 = Divide(x=w543, y=1.3) -> (x/y=w541:dbl)
            n313 = call-poly <vilib>:"WPI_RobotDriveHolonomicDrive.vi"("Rotation"=w541, "Gyro Angle"=w545, "Y"=-0.25, "X"=0.0, "RobotDriveDevRef"=w556) -> ("RobotDriveDevRef"=w555:T1)  [unwired: 4 in, 2 out]
            n314 = Greater?(x=w552, y=11.7) -> (0:w550:bool)
          }
        }
        frame #8 {
          n315 = Tick Count (ms)() -> (millisecond timer value=w560:u32)
          n316 = global write "Robot Global Data.vi" "Desired Direction"(270.0 ("Desired Direction")) -> ()
          n317 = Wait (ms)(milliseconds to wait=u32 500) -> ()  [unwired: 1 out]
          n318 = Add(x=w560, y=u32 2750) -> (x+y=w558:u32)
        }
        frame #9 {
          n319 = while {
            tunnel: w564 -> [w571]
            shift-right: [w574] -> w565
            shift-left: w566 -> [w575]
            stop <- w572 stop-if-true
            n320 = global read "Robot Global Data.vi" "Rotation"() -> (w570:dbl)
            n321 = global read "Robot Global Data.vi" "Gyro Pos"() -> (w576:dbl)
            n322 = global write "Robot Global Data.vi" "Desired Direction"(270.0 ("Desired Direction")) -> ()
            n323 = Tick Count (ms)() -> (millisecond timer value=w573:u32)
            n324 = Multiply(x=w570, y=0.6) -> (x*y=w569:dbl)
            n325 = Greater?(x=w573, y=w571) -> (0:w572:bool)
            n326 = call-poly <vilib>:"WPI_RobotDriveHolonomicDrive.vi"("Rotation"=w569, "Gyro Angle"=w576, "Y"=0.0, "X"=0.0, "RobotDriveDevRef"=w575) -> ("RobotDriveDevRef"=w574:T1)  [unwired: 4 in, 2 out]
          }
        }
        frame #10 {
          n327 = call "Drive Encoder Reset.vi"() -> ()  [unwired: 12 in]
          n328 = Wait (ms)(milliseconds to wait=u32 750) -> ()  [unwired: 1 out]
        }
        frame #11 {
          n329 = while {
            shift-right: [w583] -> w581
            shift-left: w582 -> [w593]
            stop <- w584 stop-if-true
            n330 = global read "Robot Global Data.vi" "Enc Arr G"() -> (w587:dbl)
            n331 = global read "Robot Global Data.vi" "Enc Arr D"() -> (w586:dbl)
            n332 = global read "Robot Global Data.vi" "Enc Av G"() -> (w588:dbl)
            n333 = global read "Robot Global Data.vi" "Enc Av D"() -> (w585:dbl)
            n334 = global read "Robot Global Data.vi" "Gyro Pos"() -> (w595:dbl)
            n335 = global read "Robot Global Data.vi" "Rotation"() -> (w594:dbl)
            n336 = Compound Arithmetic op=ADD(w588, w587, w586, w585) -> (w592:dbl)
            n337 = Divide(x=w592, y=4) -> (x/y=w590:dbl)
            n338 = call-poly <vilib>:"WPI_RobotDriveHolonomicDrive.vi"("Rotation"=w594, "Gyro Angle"=w595, "Y"=0.0, "X"=-0.15, "RobotDriveDevRef"=w593) -> ("RobotDriveDevRef"=w583:T1)  [unwired: 4 in, 2 out]
            n339 = Greater?(x=w590, y=0.125) -> (0:w584:bool)
          }
        }
        frame #12 {
          n340 = global write "Robot Global Data.vi" "baisser bras"(TRUE) -> ()
          n341 = call "Drive Encoder Reset.vi"() -> ()  [unwired: 12 in]
        }
        frame #13 {
          n342 = Wait (ms)(milliseconds to wait=u32 1000) -> ()  [unwired: 1 out]
        }
        frame #14 {
          n343 = while {
            tunnel: w602 -> [w612]
            stop <- w603 stop-if-true
            n344 = global read "Robot Global Data.vi" "Enc Arr G"() -> (w606:dbl)
            n345 = global read "Robot Global Data.vi" "Enc Arr D"() -> (w605:dbl)
            n346 = global read "Robot Global Data.vi" "Enc Av G"() -> (w607:dbl)
            n347 = global read "Robot Global Data.vi" "Enc Av D"() -> (w604:dbl)
            n348 = global read "Robot Global Data.vi" "Gyro Pos"() -> (w614:dbl)
            n349 = global read "Robot Global Data.vi" "Rotation"() -> (w613:dbl)
            n350 = Compound Arithmetic op=ADD(w607, w606, w605, w604) -> (w611:dbl)
            n351 = Divide(x=w611, y=4) -> (x/y=w609:dbl)
            n352 = call-poly <vilib>:"WPI_RobotDriveHolonomicDrive.vi"("Rotation"=w613, "Gyro Angle"=w614, "Y"=0.0, "X"=0.18, "RobotDriveDevRef"=w612) -> ()  [unwired: 4 in, 3 out]
            n353 = Less?(x=w609, y=-0.4) -> (x < y?=w603:bool)
          }
        }
      }
    }
    frame "Droite Niveau 3" {
      n354 = flat-sequence {
        tunnel: [w630] -> w628
        tunnel: w617 -> [w629]
        tunnel: w628 -> [w640]
        tunnel: [w640] -> w627
        tunnel: w627 -> [w642]
        tunnel: [w641] -> w626
        tunnel: w626 -> [w659]
        tunnel: [w659] -> w625
        tunnel: w625 -> [w661]
        tunnel: [w660] -> w624
        tunnel: w624 -> [w671]
        tunnel: [w671] -> w623
        tunnel: w623 -> [w673]
        tunnel: [w672] -> w622
        tunnel: w622 -> [w689]
        tunnel: [w689] -> w621
        tunnel: w621 -> [w692]
        tunnel: [w691] -> w620
        tunnel: w620 -> [w703]
        tunnel: [w702] -> w619
        tunnel: w619 -> [w720]
        tunnel: [w720] -> w618
        tunnel: w618 -> [w721]
        frame #0 {
          # "tasser a droite jusqua"
          n355 = while {
            tunnel: [w639] -> w630
            tunnel: w629 -> [w635]
            stop <- w633 stop-if-true
            n356 = global read "Robot Global Data.vi" "Enc Av G"() -> (w632:dbl)
            n357 = global read "Robot Global Data.vi" "Gyro Pos"() -> (w634:dbl)
            n358 = Greater?(x=w632, y=1500.0) -> (0:w633:bool)
            n359 = call-poly <vilib>:"WPI_RobotDriveHolonomicDrive.vi"("Rotation"=0.0, "Gyro Angle"=w634, "Y"=1.0, "X"=0.0, "RobotDriveDevRef"=w635) -> ("RobotDriveDevRef"=w639:T1)  [unwired: 4 in, 2 out]
          }
        }
        frame #1 {
          # "clean up encodeur"
          n360 = call "Drive Encoder Reset.vi"() -> ()  [unwired: 12 in]
        }
        frame #2 {
          # "avancer"
          n361 = while {
            tunnel: w642 -> [w657]
            tunnel: [w656] -> w641
            stop <- w648 stop-if-true
            n362 = global read "Robot Global Data.vi" "Enc Arr G"() -> (w645:dbl)
            n363 = global read "Robot Global Data.vi" "Enc Arr D"() -> (w644:dbl)
            n364 = global read "Robot Global Data.vi" "Enc Av G"() -> (w646:dbl)
            n365 = global read "Robot Global Data.vi" "Enc Av D"() -> (w643:dbl)
            n366 = global read "Robot Global Data.vi" "Gyro Pos"() -> (w647:dbl)
            n367 = Compound Arithmetic op=ADD(w646, w645, w644, w643) -> (w652:dbl)
            n368 = call-poly <vilib>:"WPI_RobotDriveHolonomicDrive.vi"("Rotation"=0.0, "Gyro Angle"=w647, "Y"=0.0, "X"=1.0, "RobotDriveDevRef"=w657) -> ("RobotDriveDevRef"=w656:T1)  [unwired: 4 in, 2 out]
            n369 = Divide(x=w652, y=4) -> (x/y=w650:dbl)
            n370 = Greater?(x=w650, y=42000.0) -> (0:w648:bool)
          }
        }
        frame #3 {
          n371 = global write "Robot Global Data.vi" "Desired Direction"(315.0 ("Desired Direction")) -> ()
        }
        frame #4 {
          # "rotation 45 degrer"
          n372 = while {
            tunnel: [w668] -> w660
            tunnel: w661 -> [w663]
            stop <- w665 stop-if-true
            n373 = global read "Robot Global Data.vi" "Gyro Pos"() -> (w662:dbl)
            n374 = global read "Robot Global Data.vi" "Rotation"() -> (w664:dbl)
            n375 = In Range and Coerce(upper limit=91.0, x=w662, lower limit=89.0) -> (In Range?=w665:bool)  [unwired: 1 out]
            n376 = call-poly <vilib>:"WPI_RobotDriveHolonomicDrive.vi"("Rotation"=w664, "Gyro Angle"=w662, "Y"=0.0, "X"=0.0, "RobotDriveDevRef"=w663) -> ("RobotDriveDevRef"=w668:T1)  [unwired: 4 in, 2 out]
          }
        }
        frame #5 {
          # "clean up encodeur"
          n377 = call "Drive Encoder Reset.vi"() -> ()  [unwired: 12 in]
        }
        frame #6 {
          # "avancer"
          n378 = while {
            tunnel: [w688] -> w672
            tunnel: w673 -> [w679]
            stop <- w680 stop-if-true
            n379 = global read "Robot Global Data.vi" "Enc Arr G"() -> (w676:dbl)
            n380 = global read "Robot Global Data.vi" "Enc Arr D"() -> (w675:dbl)
            n381 = global read "Robot Global Data.vi" "Enc Av G"() -> (w677:dbl)
            n382 = global read "Robot Global Data.vi" "Enc Av D"() -> (w674:dbl)
            n383 = global read "Robot Global Data.vi" "Gyro Pos"() -> (w678:dbl)
            n384 = Compound Arithmetic op=ADD(w677, w676, w675, w674) -> (w684:dbl)
            n385 = call-poly <vilib>:"WPI_RobotDriveHolonomicDrive.vi"("Rotation"=0.0, "Gyro Angle"=w678, "Y"=-0.75, "X"=0.75, "RobotDriveDevRef"=w679) -> ("RobotDriveDevRef"=w688:T1)  [unwired: 4 in, 2 out]
            n386 = Divide(x=w684, y=4) -> (x/y=w682:dbl)
            n387 = Greater?(x=w682, y=42000.0) -> (0:w680:bool)
          }
        }
        frame #7 {
          n388 = global write "Robot Global Data.vi" "Desired Direction"(0.0 ("Desired Direction")) -> ()
        }
        frame #8 {
          # "rotation jusqua 0"
          n389 = while {
            tunnel: [w699] -> w691
            tunnel: w692 -> [w694]
            stop <- w696 stop-if-true
            n390 = global read "Robot Global Data.vi" "Gyro Pos"() -> (w693:dbl)
            n391 = global read "Robot Global Data.vi" "Rotation"() -> (w695:dbl)
            n392 = In Range and Coerce(upper limit=91.0, x=w693, lower limit=89.0) -> (In Range?=w696:bool)  [unwired: 1 out]
            n393 = call-poly <vilib>:"WPI_RobotDriveHolonomicDrive.vi"("Rotation"=w695, "Gyro Angle"=w693, "Y"=0.0, "X"=0.0, "RobotDriveDevRef"=w694) -> ("RobotDriveDevRef"=w699:T1)  [unwired: 4 in, 2 out]
          }
        }
        frame #9 {
          # "se placer avec la visiom"
          n394 = while {
            tunnel: [w718] -> w702
            tunnel: w703 -> [w715]
            stop <- w716 stop-if-true
            n395 = global read "Robot Global Data.vi" "Largeur Vision"() -> (w710:dbl)
            n396 = global read "Robot Global Data.vi" "Gauche Droite Vision"() -> (w714:dbl)
            n397 = Greater?(x=w710, y=200.0) -> (0:w705:bool)
            n398 = global read "Robot Global Data.vi" "Gyro Pos"() -> (w704:dbl)
            n399 = Select(t=0.0, s=w705, f=0.6) -> (s? t:f=w708:dbl)
            n400 = In Range and Coerce(upper limit=0.08, x=w714, lower limit=-0.08) -> (In Range?=w711:bool)  [unwired: 1 out]
            n401 = call-poly <vilib>:"WPI_RobotDriveHolonomicDrive.vi"("Rotation"=0.0, "Gyro Angle"=w704, "Y"=w714, "X"=w708, "RobotDriveDevRef"=w715) -> ("RobotDriveDevRef"=w718:T1)  [unwired: 4 in, 2 out]
            n402 = And(x=w711, y=w705) -> (x .and. y?=w716:bool)
          }
        }
        frame #10 {
          # "baisser bras"
          n403 = global write "Robot Global Data.vi" "baisser bras"(TRUE) -> ()
          n404 = call "Drive Encoder Reset.vi"() -> ()  [unwired: 12 in]
        }
        frame #11 {
          # "avancer jusquaux mur"
          n405 = while {
            tunnel: w721 -> [w735]
            stop <- w727 stop-if-true
            n406 = global read "Robot Global Data.vi" "Enc Arr G"() -> (w724:dbl)
            n407 = global read "Robot Global Data.vi" "Enc Arr D"() -> (w723:dbl)
            n408 = global read "Robot Global Data.vi" "Enc Av G"() -> (w725:dbl)
            n409 = global read "Robot Global Data.vi" "Enc Av D"() -> (w722:dbl)
            n410 = global read "Robot Global Data.vi" "Gyro Pos"() -> (w726:dbl)
            n411 = Compound Arithmetic op=ADD(w725, w724, w723, w722) -> (w731:dbl)
            n412 = Divide(x=w731, y=4) -> (x/y=w729:dbl)
            n413 = call-poly <vilib>:"WPI_RobotDriveHolonomicDrive.vi"("Rotation"=0.0, "Gyro Angle"=w726, "Y"=0.0, "X"=1.0, "RobotDriveDevRef"=w735) -> ()  [unwired: 4 in, 3 out]
            n414 = Greater?(x=w729, y=42000.0) -> (0:w727:bool)
          }
        }
      }
    }
  }
